vi "sinewave_truthtable.vi"() -> ()   [LabVIEW 2018]
panel:
  out "Waveform Chart":dbl[](graph)
  out "Array":dbl[](array[numeric])
  in  "Amplitude":dbl
  in  "datapoints":i64
  in  "freq (cyc per sec)":dbl
  in  "total number of cyc":dbl
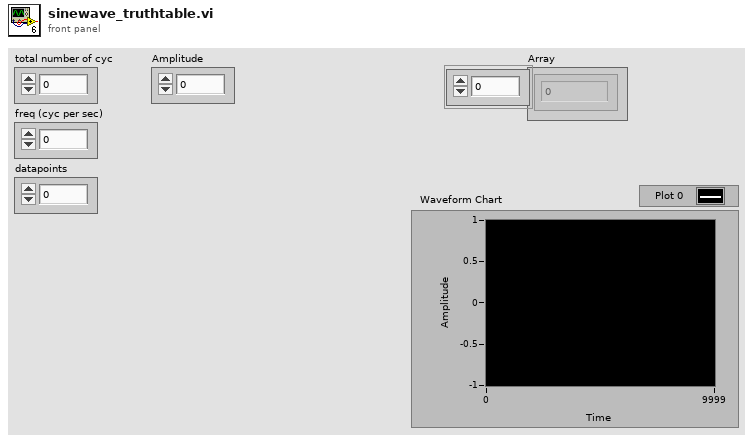
[diagram p1: front panel]
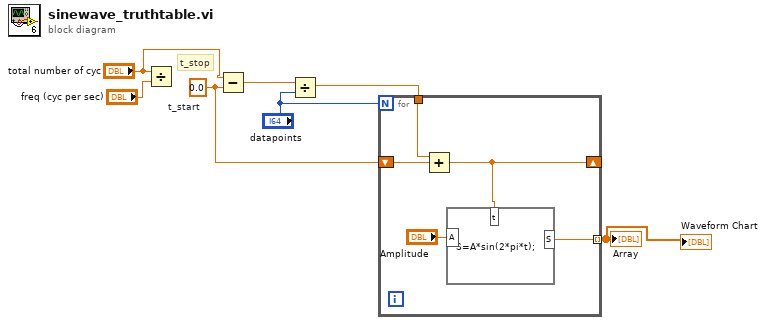
[diagram p0: block diagram]
diagram:
  w3 = 0.0  # t_start
  # "t_stop"
  n1 = Divide(x="total number of cyc", y="freq (cyc per sec)") -> ()  [unwired: 1 out]
  n2 = Subtract(x="total number of cyc", y=w3) -> (x-y=w6:dbl)
  n3 = Divide(x=w6, y="datapoints") -> (x/y=w4:dbl)
  n4 = for {
    N: "datapoints" -> [_]
    tunnel: w4 -> [w12]
    shift-right: [w8] -> _
    shift-left: w3 -> [w11]
    tunnel: [w9] -> w2 mode=indexing
    n5 = Add(x=w12, y=w11) -> (x+y=w8:dbl)
    n6 = formula code="S=A*sin(2*pi*t);"("A"="Amplitude", "t"=w8) -> ("S"=w9:dbl)
  }
  "Array" <- w2
  "Waveform Chart" <- w2
